vi "Tabor 5064 - Set Channel Load (SubVI).vi"(6 "write_delay (ms)":u32=100, 7 "GPIB Address":string="4", 8 "error_in":errorcluster, 11 "channel_loads":u32[](array[numeric])=[10000, 10000, 10000, 10000]) -> (0 "error_out":errorcluster)   [LabVIEW 2018]
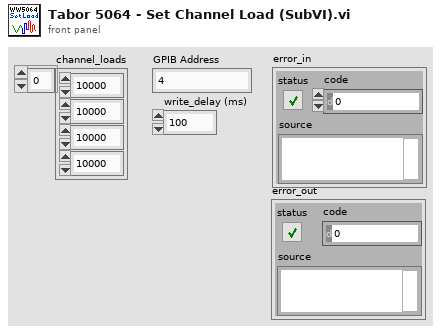
[diagram p1: front panel]
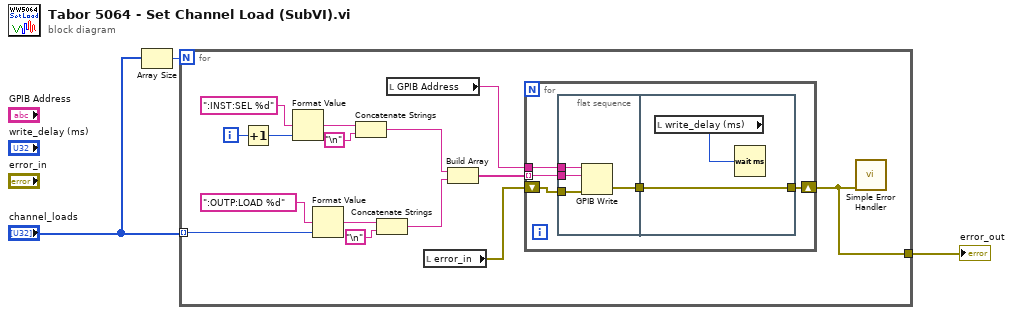
[diagram p0: block diagram]
diagram:
  n1 = Array Size(array="channel_loads") -> (size(s)=w3:i32)
  n2 = for {
    N: w3 -> [_]
    tunnel: "channel_loads" -> [w8] mode=indexing
    tunnel: [w4] -> w1
    i -> [w14]
    n3 = Increment(x=w14) -> (x+1=w17:i32)
    n4 = Format Value(format string=":INST:SEL %d", value (0)=w17) -> (output string=w18:string)  [unwired: 1 in]
    n5 = Format Value(format string=":OUTP:LOAD %d", value (0)=w8) -> (output string=w11:string)  [unwired: 1 in]
    n6 = Concatenate Strings(w18, "\n") -> (w10:string)
    n7 = Concatenate Strings(w11, "\n") -> (w9:string)
    n8 = local read "GPIB Address"() -> (w6:string)
    n9 = local read "error_in"() -> (w5:errorcluster)
    n10 = Build Array(w10, w9) -> (w7:string[])
    n11 = for {
      tunnel: w6 -> [w23]
      tunnel: w7 -> [w22] mode=indexing
      shift-right: [w21] -> w4
      shift-left: w5 -> [w20]
      n12 = flat-sequence {
        tunnel: w23 -> [w27]
        tunnel: w22 -> [w26]
        tunnel: w20 -> [w24]
        tunnel: [w25] -> w19
        tunnel: [w29] -> w21
        tunnel: w19 -> [w29]
        frame #0 {
          n13 = GPIB Write(0:w27, 1:w26, 3:w24) -> (6:w25:errorcluster)  [unwired: 2 in, 1 out]
        }
        frame #1 {
          n14 = local read "write_delay (ms)"() -> (w28:u32)
          n15 = Wait (ms)(milliseconds to wait=w28) -> ()  [unwired: 1 out]
        }
      }
    }
    n16 = call <vilib>:"Simple Error Handler.vi"("error in (no error)"=w4) -> ()  [unwired: 4 in, 5 out]
  }
  "error_out" <- w1
